vi "IPC-Core-InitializeQueues.vi"(1 "comand (Initialize)":enum16{"UnInitialize", "Initialize"}(ring), 5 "error in (no error)":errorcluster caption="错误输入（无错误）") -> (12 "6133QRef":refnum<queue>, 13 "error out":errorcluster caption="错误输出", 14 "CmdQRef":refnum<queue>, 15 "ModbusQRef":refnum<queue>, 16 "DaqQRef":refnum<queue>, 17 "DataQRef":refnum<queue>, 18 "UdpQRef":refnum<queue>, 19 "ErrorQRef":refnum<queue>)   [LabVIEW 2014]
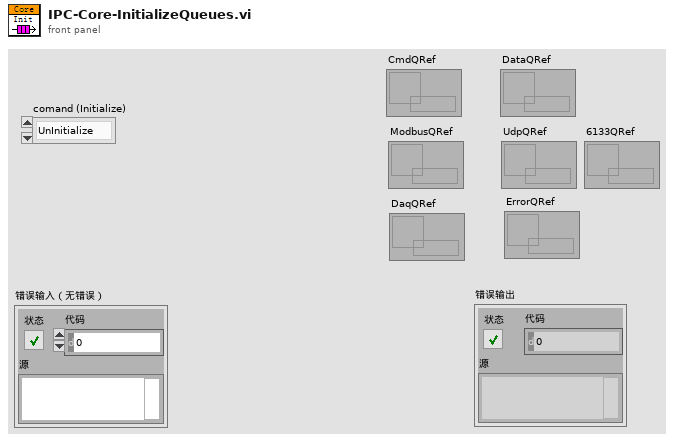
[diagram p1: front panel]
types:
  T1 = cluster{"设备名":string, "时间":timestamp, "数据":sgl[][]}
  T2 = cluster{"设备名":string, "时间":timestamp, "数据":sgl[][], "通道长度":i32[], "次数":i32}
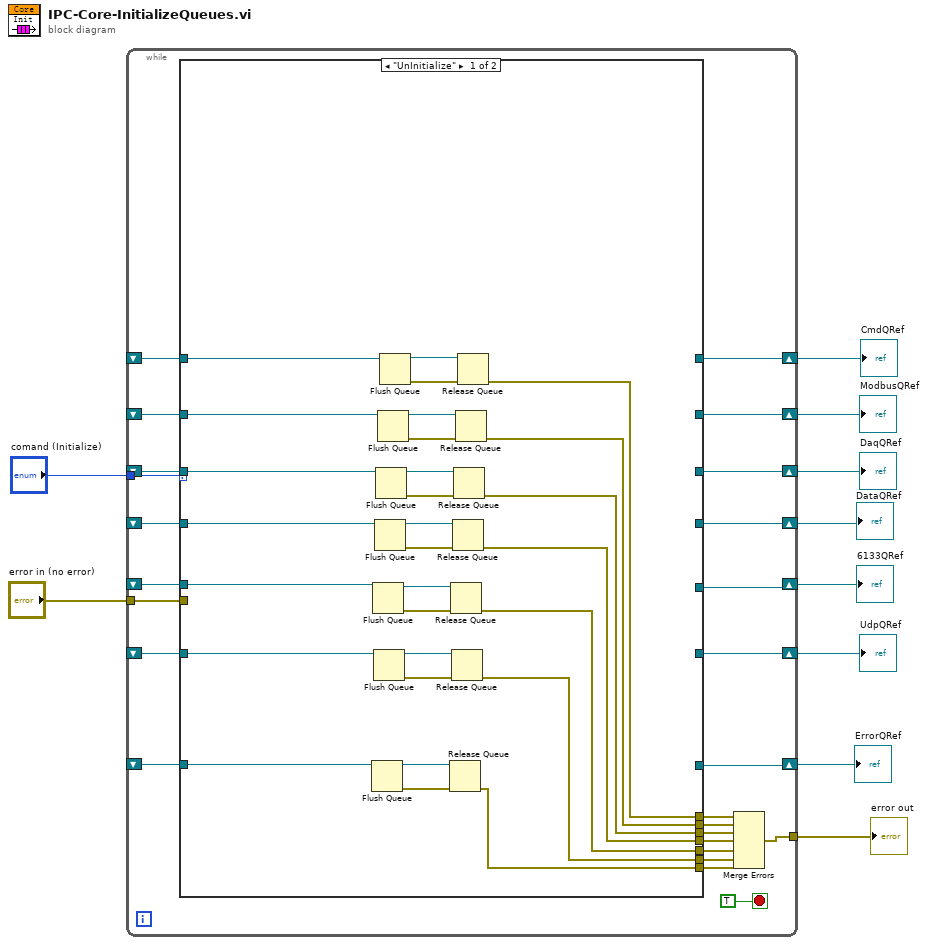
[diagram p0: block diagram]
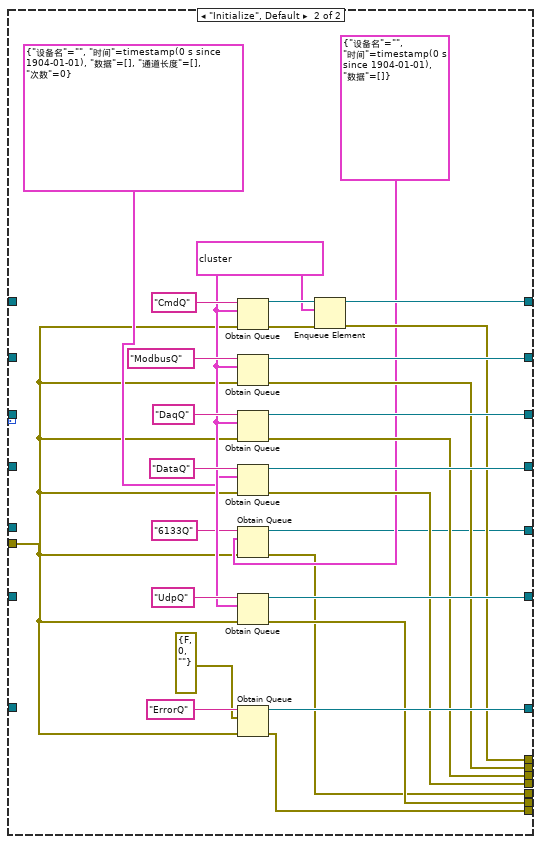
[diagram p2: hidden frame]
diagram:
  n1 = while {
    shift-right: [w34] -> w6
    shift-left: _ -> [w33]
    tunnel: "comand (Initialize)" -> [w32]
    tunnel: "error in (no error)" -> [w31]
    shift-right: [w27] -> w5
    shift-left: _ -> [w19]
    shift-right: [w28] -> w4
    shift-left: _ -> [w20]
    shift-right: [w29] -> w2
    shift-left: _ -> [w18]
    shift-right: [w30] -> w3
    shift-left: _ -> [w17]
    shift-right: [w26] -> w7
    shift-left: _ -> [w16]
    tunnel: [w21] -> w8
    shift-right: [w12] -> w1
    shift-left: _ -> [w11]
    stop <- TRUE stop-if-true
    n2 = case shown="\"UnInitialize\"" w32 {
      tunnel: [_ w89] -> w34
      tunnel: w33 -> [w51 _]
      tunnel: w31 -> [_ w66]
      tunnel: [_ w80] -> w30
      tunnel: [_ w79] -> w29
      tunnel: [_ w78] -> w28
      tunnel: [_ w77] -> w27
      tunnel: [_ w76] -> w26
      tunnel: [w40 w75] -> w25
      tunnel: [w41 w74] -> w24
      tunnel: [w42 w72] -> w23
      tunnel: [w43 w71] -> w22
      tunnel: [w44 w70] -> w14
      tunnel: [w45 w73] -> w13
      tunnel: w20 -> [w49 _]
      tunnel: w19 -> [w50 _]
      tunnel: w18 -> [w48 _]
      tunnel: w17 -> [w47 _]
      tunnel: w16 -> [w46 _]
      tunnel: [_ w65] -> w12
      tunnel: [w36 w64] -> w15
      tunnel: w11 -> [w37 _]
      frame "UnInitialize" {
        n3 = Flush Queue(queue=w46) -> (queue out=w53:refnum<queue>, error out=w52:errorcluster)  [unwired: 1 in, 1 out]
        n4 = Flush Queue(queue=w37) -> (queue out=w38:refnum<queue>, error out=w39:errorcluster)  [unwired: 1 in, 1 out]
        n5 = Flush Queue(queue=w47) -> (queue out=w55:refnum<queue>, error out=w54:errorcluster)  [unwired: 1 in, 1 out]
        n6 = Flush Queue(queue=w48) -> (queue out=w57:refnum<queue>, error out=w56:errorcluster)  [unwired: 1 in, 1 out]
        n7 = Flush Queue(queue=w49) -> (queue out=w59:refnum<queue>, error out=w58:errorcluster)  [unwired: 1 in, 1 out]
        n8 = Flush Queue(queue=w50) -> (queue out=w61:refnum<queue>, error out=w60:errorcluster)  [unwired: 1 in, 1 out]
        n9 = Flush Queue(queue=w51) -> (queue out=w63:refnum<queue>, error out=w62:errorcluster)  [unwired: 1 in, 1 out]
        n10 = Release Queue(queue=w53, error in (no error)=w52) -> (error out=w45:errorcluster)  [unwired: 1 in, 2 out]
        n11 = Release Queue(queue=w38, error in (no error)=w39) -> (error out=w36:errorcluster)  [unwired: 1 in, 2 out]
        n12 = Release Queue(queue=w55, error in (no error)=w54) -> (error out=w44:errorcluster)  [unwired: 1 in, 2 out]
        n13 = Release Queue(queue=w57, error in (no error)=w56) -> (error out=w43:errorcluster)  [unwired: 1 in, 2 out]
        n14 = Release Queue(queue=w59, error in (no error)=w58) -> (error out=w42:errorcluster)  [unwired: 1 in, 2 out]
        n15 = Release Queue(queue=w61, error in (no error)=w60) -> (error out=w41:errorcluster)  [unwired: 1 in, 2 out]
        n16 = Release Queue(queue=w63, error in (no error)=w62) -> (error out=w40:errorcluster)  [unwired: 1 in, 2 out]
      }
      frame "Initialize", Default {
        w83 = cluster{variant, string} {variant, "Cmd::Initialize"}
        n17 = Obtain Queue(name (unnamed)="CmdQ" ("名称（未命名）"), element data type=w83, error in (no error)=w66) -> (queue out=w90:refnum<queue>, error out=w81:errorcluster)  [unwired: 2 in, 1 out]
        n18 = Obtain Queue(name (unnamed)="ModbusQ" ("名称（未命名）"), element data type=w83, error in (no error)=w66) -> (queue out=w77:refnum<queue>, error out=w74:errorcluster)  [unwired: 2 in, 1 out]
        n19 = Obtain Queue(name (unnamed)="DaqQ" ("名称（未命名）"), element data type=w83, error in (no error)=w66) -> (queue out=w78:refnum<queue>, error out=w72:errorcluster)  [unwired: 2 in, 1 out]
        n20 = Obtain Queue(name (unnamed)="DataQ" ("名称（未命名）"), element data type=T2 {"设备名"="", "时间"=timestamp(0 s since 1904-01-01), "数据"=[], "通道长度"=[], "次数"=0}, error in (no error)=w66) -> (queue out=w79:refnum<queue>, error out=w71:errorcluster)  [unwired: 2 in, 1 out]
        n21 = Obtain Queue(name (unnamed)="6133Q" ("名称（未命名）"), element data type=T1 {"设备名"="", "时间"=timestamp(0 s since 1904-01-01), "数据"=[]}, error in (no error)=w66) -> (queue out=w65:refnum<queue>, error out=w64:errorcluster)  [unwired: 2 in, 1 out]
        n22 = Obtain Queue(name (unnamed)="UdpQ" ("名称（未命名）"), element data type=w83, error in (no error)=w66) -> (queue out=w80:refnum<queue>, error out=w70:errorcluster)  [unwired: 2 in, 1 out]
        n23 = Obtain Queue(name (unnamed)="ErrorQ" ("名称（未命名）"), element data type=errorcluster {"status"=FALSE, "code"=0, "source"=""} ("错误常量"), error in (no error)=w66) -> (queue out=w76:refnum<queue>, error out=w73:errorcluster)  [unwired: 2 in, 1 out]
        n24 = Enqueue Element(queue=w90, element=w83, error in (no error)=w81) -> (queue out=w89:refnum<queue>, error out=w75:errorcluster)  [unwired: 1 in, 1 out]
      }
    }
    n25 = Merge Errors(w25, w24, w23, w22, w15, w14, w13) -> (w21:errorcluster)
  }
  "error out" <- w8
  "ErrorQRef" <- w7
  "CmdQRef" <- w6
  "ModbusQRef" <- w5
  "DaqQRef" <- w4
  "UdpQRef" <- w3
  "DataQRef" <- w2
  "6133QRef" <- w1
